vi "Search in DB.vi"(8 "error in (no error)":errorcluster, 11 "DB Data in":T1 {"Balance" format="%.2f"; "Account" format="%05d"}) -> (0 "error out":errorcluster, 1 "Index":i64, 2 "DB Record":T3 {"Balance" format="%.2f"; "Account" format="%05d"}, 3 "refnum out":refnum<file>)   [LabVIEW 2017]
uses:
  Type Definitions/DB Record.ctl
  Type Definitions/DB Data.ctl
  Type Definitions/DB Info.ctl
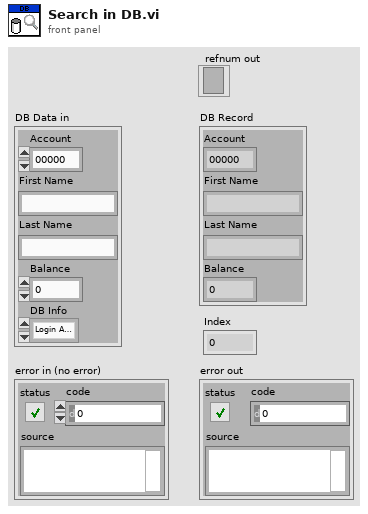
[diagram p1: front panel]
types:
  T1 = typedef "DB Data.ctl" = cluster{"Account":i32, "First Name":string, "Last Name":string, "Balance":fxp<+/-,64,35>, "DB Info":T2}
  T2 = typedef "DB Info.ctl" = enum16{"Login Accepted", "Invalid Login", "Deposit Complete", "Withdrawal Complete", "Withdrawal Failed", "Terminate"}
  T3 = typedef "DB Record.ctl" = cluster{"Account":i32, "First Name":string, "Last Name":string, "Balance":fxp<+/-,64,35>}
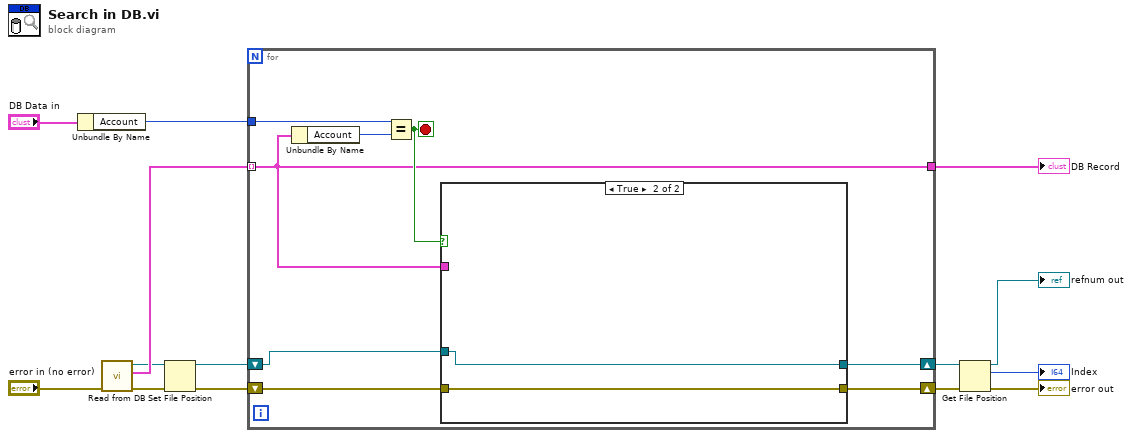
[diagram p0: block diagram]
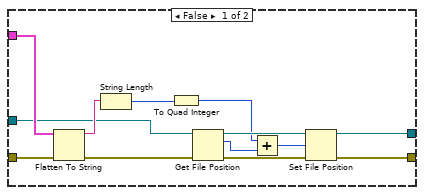
[diagram p2: hidden frame]
diagram:
  n1 = Unbundle By Name("DB Data in") -> ("Account"=w12:i32)
  n2 = call "Read from DB.vi"("error in (no error)"="error in (no error)") -> ("error out"=w9:errorcluster, "Array"=w10:T3[], "refnum out"=w8:refnum<file>)  [unwired: 8 in]
  n3 = Set File Position(refnum=w8, error in=w9) -> (refnum out=w6:refnum<file>, error out=w7:errorcluster)  [unwired: 2 in]
  n4 = for {
    tunnel: w10 -> [w17] mode=indexing
    tunnel: w12 -> [w22]
    tunnel: [w17] -> w11
    shift-right: [w18] -> w5
    shift-left: w7 -> [w19]
    shift-right: [w15] -> w4
    shift-left: w6 -> [w16]
    stop <- w20 stop-if-true
    n5 = Unbundle By Name(w17) -> ("Account"=w21:i32)
    n6 = Equal?(x=w22, y=w21) -> (x = y?=w20:bool)
    n7 = case shown="True" w20 {
      tunnel: w19 -> [w35 w37]
      tunnel: [w32 w37] -> w18
      tunnel: w17 -> [w34 _]
      tunnel: w16 -> [w31 w36]
      tunnel: [w25 w36] -> w15
      frame False {
        n8 = Flatten To String(anything=w34, error in (no error)=w35) -> (data string=w33:string, error out=w30:errorcluster)  [unwired: 2 in, 1 out]
        n9 = String Length(string=w33) -> (length=w24:i32)
        n10 = To Quad Integer(1:w24) -> (0:w23:i64)
        n11 = Get File Position(4:w30, 7:w31) -> (0:w29:errorcluster, 2:w27:i64, 3:w28:refnum<file>)
        n12 = Add(x=w23, y=w27) -> (x+y=w26:i64)
        n13 = Set File Position(offset (in bytes) (0)=w26, refnum=w28, error in=w29) -> (refnum out=w25:refnum<file>, error out=w32:errorcluster)  [unwired: 1 in]
      }
      frame True {
      }
    }
  }
  "DB Record" <- w11
  n14 = Get File Position(4:w5, 7:w4) -> (0:→"error out":errorcluster, 2:→"Index":i64, 3:→"refnum out":refnum<file>)
